vi "excavator2D_with_supplied_X.vi"() -> ()   [LabVIEW 2013]
panel:
  in  "Temperature sorted":dbl[](array[numeric])=[0.0799849, 0.09042059630155563, 0.09053420275449753, 0.0994160994887352, 0.10036399960517883, 0.10981100052595139, 0.11162599921226501, 0.12009900063276291, 0.12036000192165375, 0.13899199664592743, 0.14191600680351257, 0.1584939956665039, 0.160862997174263, 0.17834900319576263, 0.18172399699687958, 0.19769799709320068, 0.20004400610923767, 0.22258999943733215, 0.23762699961662292, 0.24158400297164917, 0.2644129991531372, 0.280009001493454, 0.2801539897918701, 0.30009400844573975, 0.3009060025215149, 0.3088909983634949]
  in  "Phase":dbl[][](graph)=array26x201[5226 elements]
  in  "Tab Control":enum32{"Page 1", "Page 2"}(tab)
  in  "Limits":bool
  in  "Name":string="tiBridge_newSample_phase_raw"
  in  "y Min":dbl=2.0 format="%#_13g"
  in  "y Max":dbl=16.0 format="%#_13g"
  in  "?":bool
  in  "Ring":u16(ring) items=["Windows", "Mac"]
  in  "Transpose?":bool
  out "Match":bool=TRUE
  out "yPoints":i32=201
  out "xPoints":i32=26
  # "1) Takes in a 2D image\n    a set of X values and\n    a range for y Values\n\n2) Creates a file:\n#no_x by no_y\nx1 y1 z1\nx1 y2 z2\nx1 y3 z3\n...\nx4 y1 z?"
  # "Data on graph"
  # "All Data"
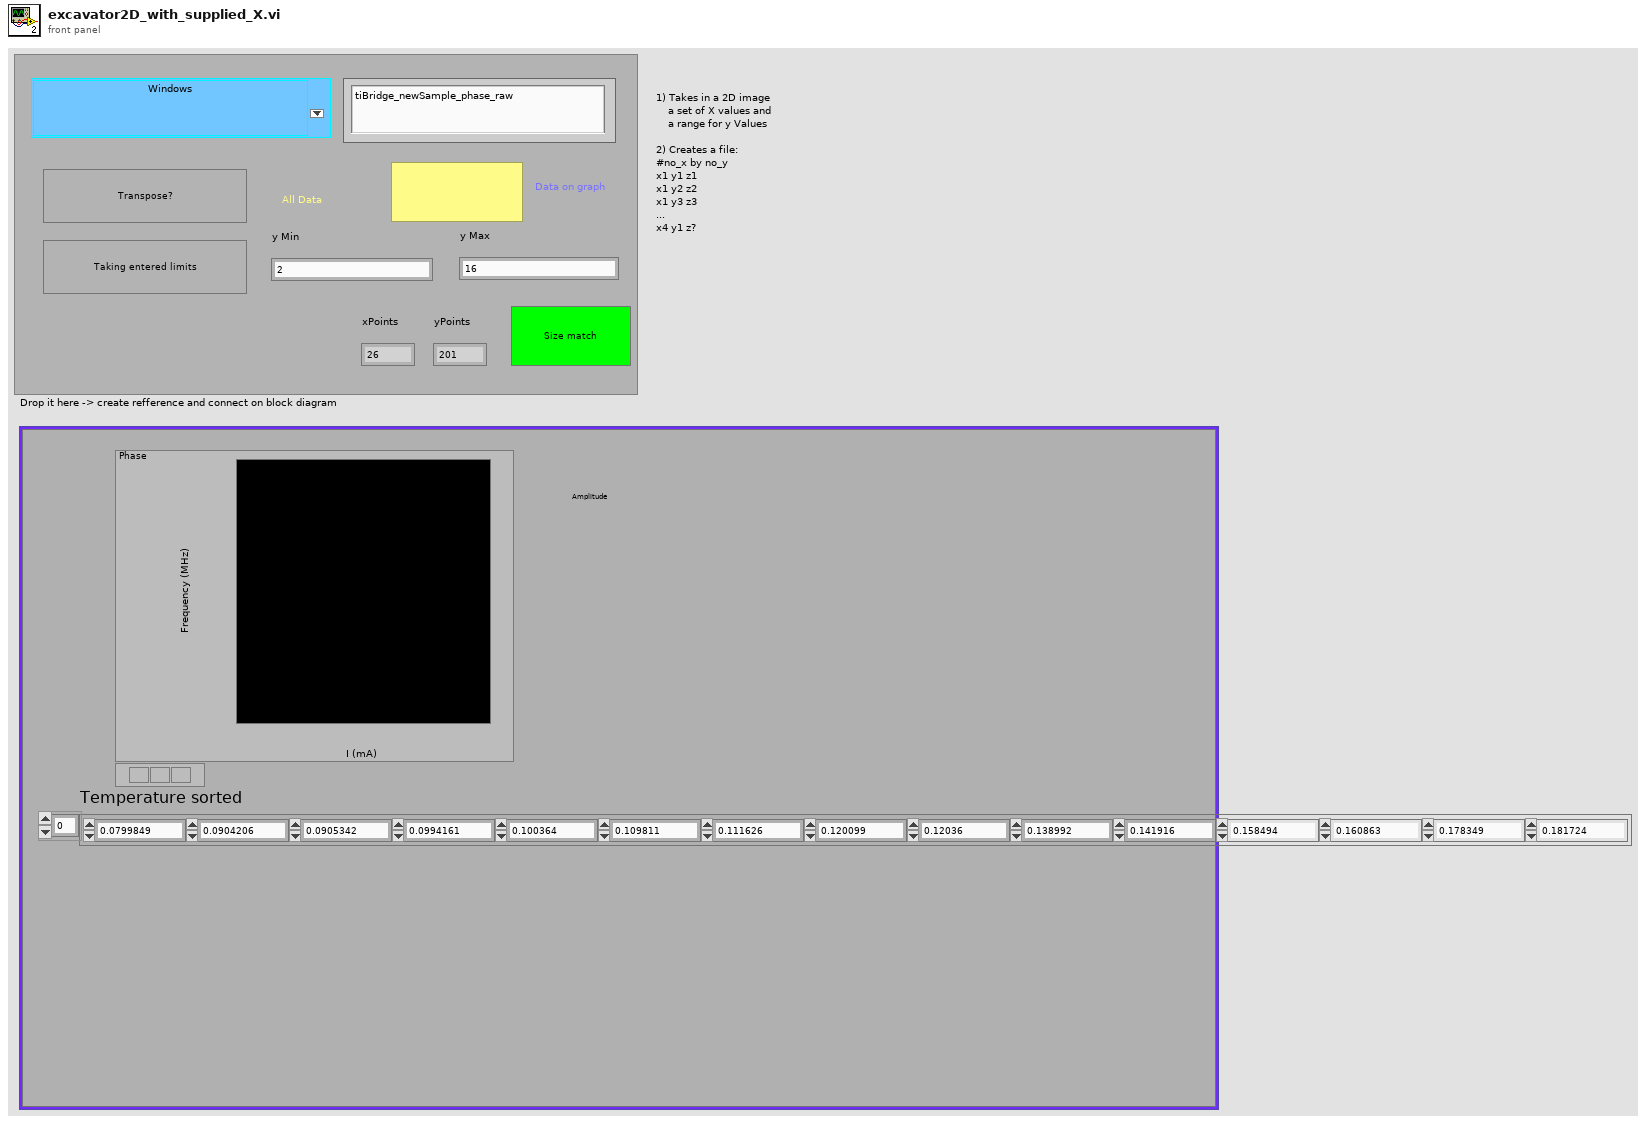
[diagram p1: front panel]
types:
  T1 = enum16{"open", "replace", "create", "open or create", "replace or create", "replace or create with confirmation"}
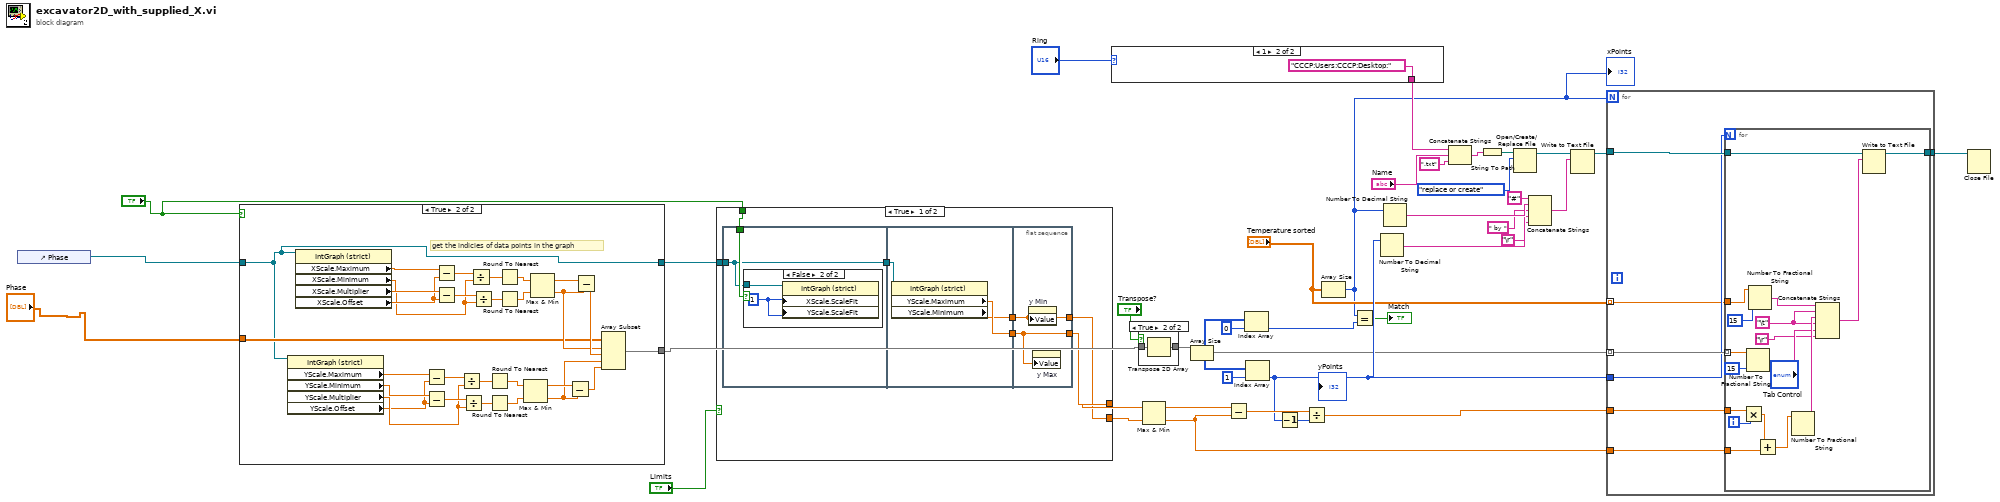
[diagram p0: block diagram]
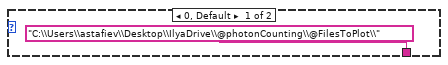
[diagram p3: hidden frame]
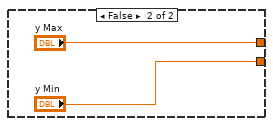
[diagram p6: hidden frame]
diagram:
  n1 = control-ref of="Phase"() -> (w9:refnum<vi>)
  n2 = case shown="True" "?" {
    tunnel: "Phase" -> [w41 w49]
    tunnel: w9 -> [w40 w42]
    tunnel: [w41 w43] -> w6
    tunnel: [w40 w42] -> w28
    frame False {
    }
    frame True {
      # "get the indicies of data points in the graph"
      n3 = property class="IntGraph (strict)"(reference=w42) -> ("YScale.Maximum"=w58:dbl, "YScale.Minimum"=w57:dbl, "YScale.Multiplier"=w56:dbl, "YScale.Offset"=w55:dbl)  [unwired: 1 in, 2 out]
      n4 = property class="IntGraph (strict)"(reference=w42) -> ("XScale.Maximum"=w67:dbl, "XScale.Minimum"=w70:dbl, "XScale.Multiplier"=w63:dbl, "XScale.Offset"=w64:dbl)  [unwired: 1 in, 2 out]
      n5 = Subtract(x=w58, y=w55) -> (x-y=w60:dbl)
      n6 = Subtract(x=w57, y=w55) -> (x-y=w59:dbl)
      n7 = Subtract(x=w67, y=w64) -> (x-y=w68:dbl)
      n8 = Subtract(x=w70, y=w64) -> (x-y=w69:dbl)
      n9 = Divide(x=w60, y=w56) -> (x/y=w61:dbl)
      n10 = Divide(x=w59, y=w56) -> (x/y=w62:dbl)
      n11 = Divide(x=w68, y=w63) -> (x/y=w66:dbl)
      n12 = Divide(x=w69, y=w63) -> (x/y=w65:dbl)
      n13 = Round To Nearest(number=w61) -> (nearest integer value=w47:dbl)
      n14 = Round To Nearest(number=w62) -> (nearest integer value=w46:dbl)
      n15 = Round To Nearest(number=w66) -> (nearest integer value=w54:dbl)
      n16 = Round To Nearest(number=w65) -> (nearest integer value=w53:dbl)
      n17 = Max & Min(x=w47, y=w46) -> (max(x,y)=w48:dbl, min(x,y)=w44:dbl)
      n18 = Max & Min(x=w54, y=w53) -> (max(x,y)=w51:dbl, min(x,y)=w50:dbl)
      n19 = Subtract(x=w48, y=w44) -> (x-y=w45:dbl)
      n20 = Subtract(x=w51, y=w50) -> (x-y=w52:dbl)
      n21 = Array Subset(array=w49, index (row)=w50, length (row)=w52, index (col)=w44, length (col)=w45) -> (w43:dbl[][])
    }
  }
  n22 = case shown="True" "Limits" {
    tunnel: [w76 "y Max"] -> w26
    tunnel: [w75 "y Min"] -> w25
    tunnel: w28 -> [w77 _]
    tunnel: "?" -> [w73 _]
    frame True {
      n23 = flat-sequence {
        tunnel: w77 -> [w78]
        tunnel: [w78] -> w74
        tunnel: w73 -> [w79]
        tunnel: w74 -> [w84]
        tunnel: [w83] -> w72
        tunnel: [w82] -> w71
        tunnel: [w85] -> w75
        tunnel: [w86] -> w76
        tunnel: w72 -> [w86]
        tunnel: w71 -> [w85]
        frame #0 {
          n24 = case shown="False" w79 {
            tunnel: w78 -> [_ w80]
            frame True {
            }
            frame False {
              w81 = u8 1 ("X Scale.Scale Fit")
              n25 = property class="IntGraph (strict)"(reference=w80, "XScale.ScaleFit"=w81, "YScale.ScaleFit"=w81) -> ()  [unwired: 1 in, 2 out]
            }
          }
        }
        frame #1 {
          n26 = property class="IntGraph (strict)"(reference=w84) -> ("YScale.Maximum"=w83:dbl, "YScale.Minimum"=w82:dbl)  [unwired: 1 in, 2 out]
        }
        frame #2 {
          n27 = property on="y Min" class="DigNum (strict)"("Value"=w85) -> ()  [unwired: 2 in, 2 out]
          n28 = property on="y Max" class="DigNum (strict)"("Value"=w86) -> ()  [unwired: 2 in, 2 out]
        }
      }
    }
    frame False {
    }
  }
  n29 = case shown="1" "Ring" {
    tunnel: ["C:\\Users\\astafiev\\Desktop\\IlyaDrive\\@photonCounting\\@FilesToPlot\\" ("Directory") "CCCP:Users:CCCP:Desktop:" ("Directory")] -> w11
    frame 0, Default {
    }
    frame 1 {
    }
  }
  n30 = case shown="True" "Transpose?" {
    tunnel: w6 -> [w91 w93]
    tunnel: [w91 w92] -> w7
    frame False {
    }
    frame True {
      n31 = Transpose 2D Array(2D array=w93) -> (transposed array=w92:dbl[][])
    }
  }
  n32 = Max & Min(x=w26, y=w25) -> (max(x,y)=w23:dbl, min(x,y)=w24:dbl)
  n33 = Array Size(array=w7) -> (size(s)=w29:i32[])
  n34 = Subtract(x=w23, y=w24) -> (x-y=w31:dbl)
  n35 = Index Array(array=w29, index=0) -> (element=w2:i32)
  n36 = Index Array(array=w29, index=1) -> (element=w14:i32)
  "yPoints" <- w14
  n37 = Decrement(x=w14) -> (x-1=w22:i32)
  n38 = Divide(x=w31, y=w22) -> (x/y=w34:dbl)
  n39 = Array Size(array="Temperature sorted") -> (size(s)=w3:i32)
  "xPoints" <- w3
  n40 = Equal?(x=w3, y=w2) -> (x = y?=→"Match":bool)
  n41 = Number To Decimal String(number=w14) -> (decimal integer string=w18:string)  [unwired: 1 in]
  n42 = Number To Decimal String(number=w3) -> (decimal integer string=w20:string)  [unwired: 1 in]
  n43 = Concatenate Strings(w11, "Name", ".txt" ("FileName 2")) -> (w39:string)
  n44 = String To Path(string=w39) -> (path=w38:path)
  n45 = Open/Create/Replace File(file path (use dialog)=w38, operation (0:open)=T1."replace or create") -> (refnum out=w16:refnum<file>)  [unwired: 4 in, 2 out]
  n46 = Concatenate Strings("#" ("string"), w20, " by " ("string"), w18, "\r") -> (w17:string)
  n47 = Write to Text File(file (use dialog)=w16, text=w17) -> (refnum out=w15:refnum<file>)  [unwired: 2 in, 2 out]
  n48 = for {
    N: w3 -> [_]
    tunnel: w7 -> [w100] mode=indexing
    tunnel: w15 -> [w99]
    tunnel: w24 -> [w98]
    tunnel: w34 -> [w97]
    tunnel: [w96] -> w33
    tunnel: w14 -> [w95]
    tunnel: "Temperature sorted" -> [w94] mode=indexing
    n49 = for {
      N: w95 -> [_]
      tunnel: w100 -> [w112] mode=indexing
      tunnel: w99 -> [w117]
      tunnel: w98 -> [w113]
      tunnel: w97 -> [w115]
      tunnel: w94 -> [w111]
      tunnel: [w103] -> w96
      i -> [w114]
      w106 = "\t"
      n50 = Multiply(x=w115, y=w114) -> (x*y=w116:dbl)
      n51 = Number To Fractional String(number=w112, precision (6)=i16 15) -> (F-format string=w107:string)  [unwired: 2 in]
      n52 = Number To Fractional String(number=w111, precision (6)=i16 15) -> (F-format string=w110:string)  [unwired: 2 in]
      n53 = Add(x=w116, y=w113) -> (x+y=w109:dbl)
      n54 = Number To Fractional String(number=w109) -> (F-format string=w108:string)  [unwired: 3 in]
      n55 = Concatenate Strings(w110, w106, w108, w106, w107, "\r") -> (w104:string)
      n56 = Write to Text File(file (use dialog)=w117, text=w104) -> (refnum out=w103:refnum<file>)  [unwired: 2 in, 2 out]
    }
  }
  n57 = Close File(refnum=w33) -> ()  [unwired: 1 in, 2 out]
